vi "tree.vi"(8 "错误输入（无错误）":errorcluster, 11 "search":refnum<vi>) -> (0 "error out":errorcluster, 3 "引用输出":refnum<vi>)   [LabVIEW 2018]
uses:
  Global.vi
  <vilib>/Instr/_visa.llb/VISA Find Search Mode.ctl
panel:
  out "路径":path
  in  "Comunication ports":string(tree)="APMDAQ::0x06"
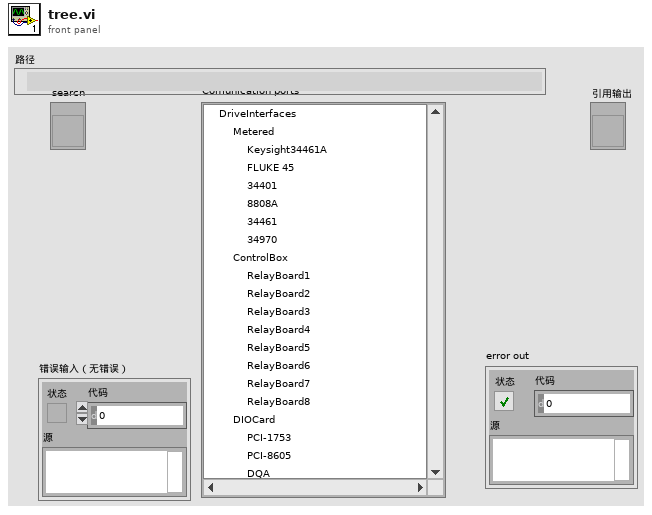
[diagram p1: front panel]
types:
  T1 = enum32{"invalid app kind", "Development System", "Run Time System", "Student Edition", "Embedded LabVIEW", "Evaluation", "Custom"}
  T2 = typedef "imagedata.ctl" = cluster{"image type":i32, "image depth":i32, "image":u8[], "mask":u8[], "colors":u32[], "Rectangle":cluster{"left":i16, "top":i16, "right":i16, "bottom":i16}}
  T3 = typedef "VISA Find Search Mode.ctl" = u32
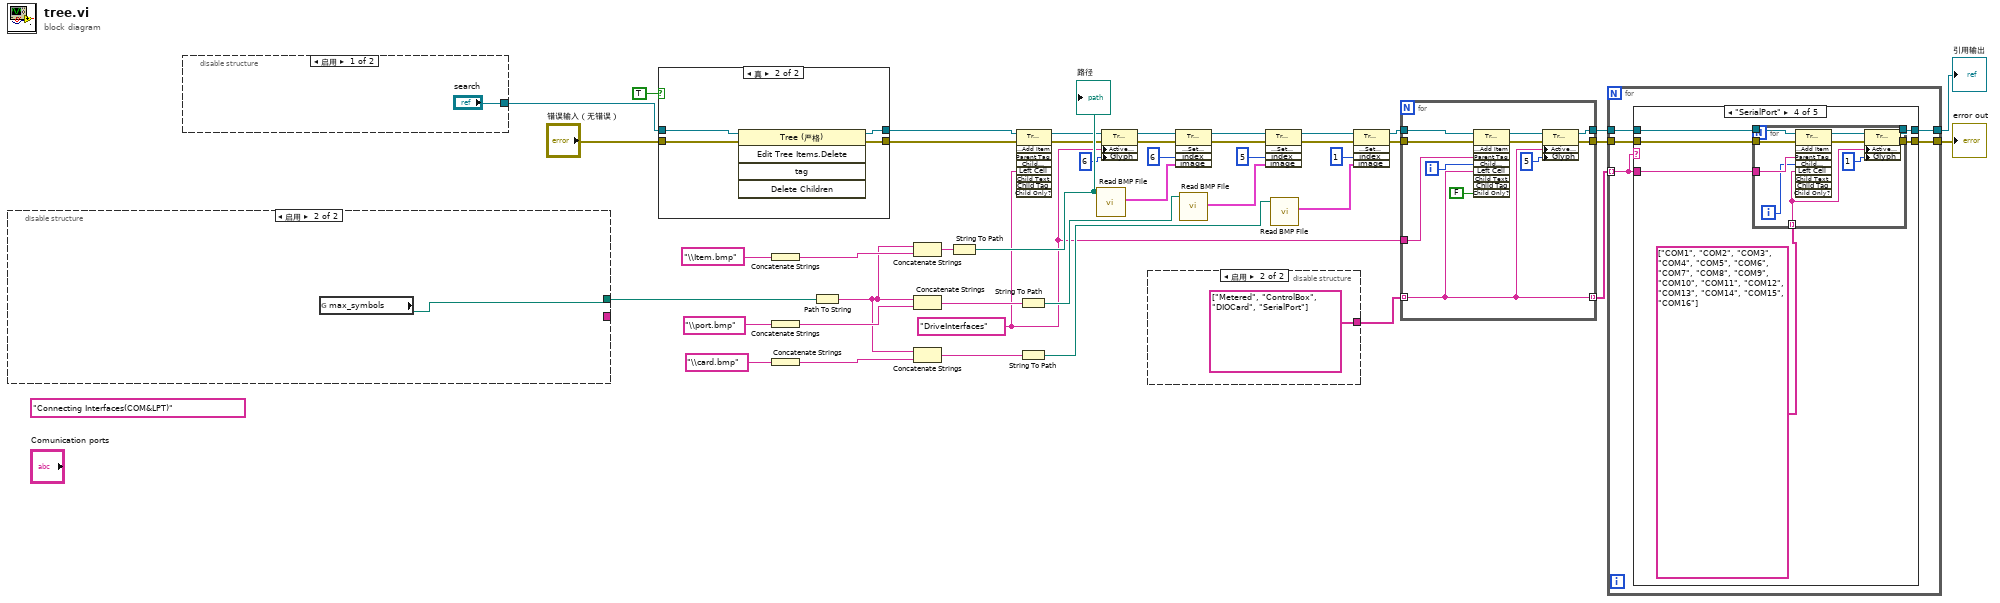
[diagram p0: block diagram]
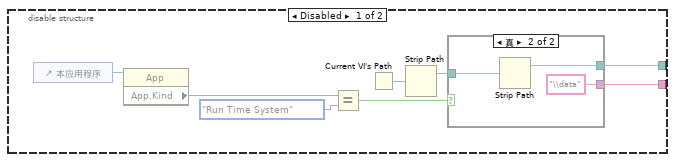
[diagram p2: hidden frame]
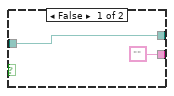
[diagram p3: hidden frame]
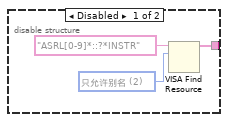
[diagram p4: hidden frame]
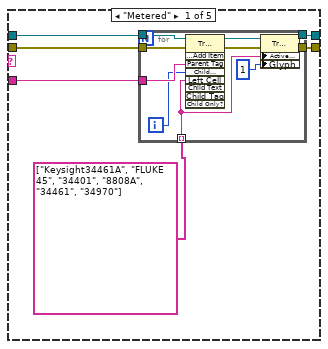
[diagram p5: hidden frame]
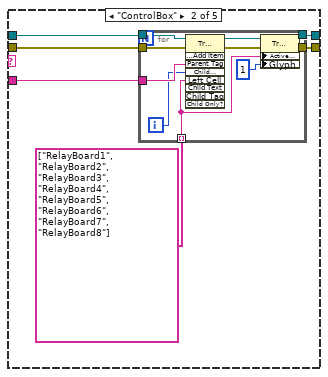
[diagram p6: hidden frame]
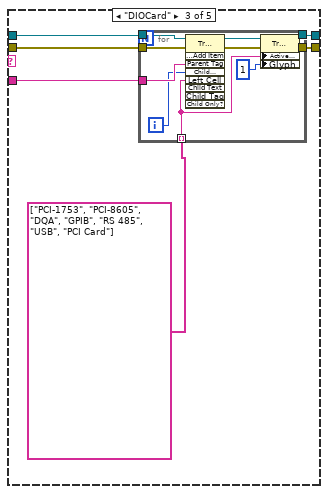
[diagram p7: hidden frame]
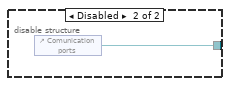
[diagram p10: hidden frame]
diagram:
  w3 = "DriveInterfaces" ("父项标识符")
  (unwired) "Connecting Interfaces(COM&LPT)" ("父项标识符")
  n1 = disable-structure shown="启用" {
    disable-tunnel: [w51 w57] -> w41
    disable-tunnel: [w44 _] -> _
    frame Disabled {
      n2 = control-ref of="本应用程序"() -> (w45:refnum<vi>)
      n3 = property class="App"(reference=w45) -> ("App.Kind"=w46:T1)  [unwired: 1 in, 2 out]
      n4 = Equal?(x=w46, y=T1."Run Time System" ("应用程序:类别")) -> (x = y?=w48:bool)
      n5 = Current VI's Path() -> (path=w49:path)
      n6 = Strip Path(path=w49) -> (stripped path=w50:path)  [unwired: 1 out]
      n7 = case shown="真" w48 {
        tunnel: w50 -> [w53 w56]
        tunnel: [w53 w55] -> w51
        tunnel: ["" "\\data"] -> w44
        frame False {
        }
        frame True {
          n8 = Strip Path(path=w56) -> (stripped path=w55:path)  [unwired: 1 out]
        }
      }
    }
    frame Enabled {
      n9 = global read "Global.vi" "max_symbols"() -> (w57:path)
    }
  }
  n10 = disable-structure shown="启用" {
    disable-tunnel: ["search" w59] -> w35
    frame Enabled {
    }
    frame Disabled {
      n11 = control-ref of="Comunication ports"() -> (w59:refnum<vi>)
    }
  }
  n12 = case shown="真" TRUE {
    tunnel: "错误输入（无错误）" -> [w60 w65]
    tunnel: [w60 w64] -> w37
    tunnel: [w61 w63] -> w22
    tunnel: w35 -> [w61 w62]
    frame False {
    }
    frame True {
      n13 = invoke class="Tree (严格)" method="Edit Tree Items.Delete"(reference=w62, error in=w65) -> (reference out=w63:refnum<vi>, error out=w64:errorcluster)  [unwired: 3 in, 3 out]
    }
  }
  n14 = Concatenate Strings("\\Item.bmp") -> (w33:string)
  n15 = Concatenate Strings("\\port.bmp") -> (w42:string)
  n16 = Concatenate Strings("\\card.bmp") -> (w43:string)
  n17 = Path To String(path=w41) -> (string=w32:string)
  n18 = Concatenate Strings(w32, w33) -> (w31:string)
  n19 = Concatenate Strings(w32, w42) -> (w39:string)
  n20 = Concatenate Strings(w32, w43) -> (w40:string)
  n21 = String To Path(string=w31) -> (path=w23:path)
  "路径" <- w23
  n22 = invoke class="Tree (严格)" method="Edit Tree Items.Add Item"(reference=w22, error in=w37, "Left Cell"=w3) -> (reference out=w18:refnum<vi>, error out=w19:errorcluster)  [unwired: 6 in, 7 out]
  n23 = String To Path(string=w39) -> (path=w27:path)
  n24 = String To Path(string=w40) -> (path=w28:path)
  n25 = call <vilib>:"Read BMP File.vi"("path to BMP file"=w23) -> ("image data"=w24:T2)  [unwired: 1 in, 9 out]
  n26 = property class="Tree (严格)"(reference=w18, error in=w19, "Active Item Tag"=w3, "Glyph"=6 ("活动项:符号索引")) -> (reference out=w8:refnum<vi>, error out=w7:errorcluster)
  n27 = disable-structure shown="启用" {
    disable-tunnel: [w68 string[] ["Metered", "ControlBox", "DIOCard", "SerialPort"] ("find list")] -> w21
    frame Disabled {
      w67 = T3 2 items=["仅允许规范名称"=0, "只允许别名"=2, "包含匹配别名"=3, "包含所有别名"=4] ("Search Mode")
      n28 = VISA Find Resource(10:w67, 11:"ASRL[0-9]*::?*INSTR" ("表达式(\"?*\")")) -> (3:w68:string[])  [unwired: 1 in, 2 out]
    }
    frame Enabled {
    }
  }
  n29 = invoke class="Tree (严格)" method="Custom Item Symbols.Set Symbol"(reference=w8, error in=w7, "index"=6 ("索引"), "image"=w24) -> (reference out=w6:refnum<vi>, error out=w5:errorcluster)  [unwired: 1 in, 3 out]
  n30 = call <vilib>:"Read BMP File.vi"("path to BMP file"=w27) -> ("image data"=w25:T2)  [unwired: 1 in, 9 out]
  n31 = invoke class="Tree (严格)" method="Custom Item Symbols.Set Symbol"(reference=w6, error in=w5, "index"=5 ("索引"), "image"=w25) -> (reference out=w12:refnum<vi>, error out=w13:errorcluster)  [unwired: 1 in, 3 out]
  n32 = call <vilib>:"Read BMP File.vi"("path to BMP file"=w28) -> ("image data"=w26:T2)  [unwired: 1 in, 9 out]
  n33 = invoke class="Tree (严格)" method="Custom Item Symbols.Set Symbol"(reference=w12, error in=w13, "index"=1 ("索引"), "image"=w26) -> (reference out=w14:refnum<vi>, error out=w15:errorcluster)  [unwired: 1 in, 3 out]
  n34 = for {
    tunnel: [w74] -> w11
    tunnel: w3 -> [w79]
    tunnel: w21 -> [w70] mode=indexing
    tunnel: w14 -> [w77]
    tunnel: w15 -> [w76]
    tunnel: [w71] -> w10
    tunnel: [w70] -> w9 mode=indexing
    i -> [w78]
    n35 = invoke class="Tree (严格)" method="Edit Tree Items.Add Item"(reference=w77, error in=w76, "Parent Tag"=w79, "Child Position"=w78, "Left Cell"=w70, "Child Only?"=FALSE ("仅作为子项？")) -> (reference out=w75:refnum<vi>, error out=w73:errorcluster)  [unwired: 3 in, 7 out]
    n36 = property class="Tree (严格)"(reference=w75, error in=w73, "Active Item Tag"=w70, "Glyph"=5 ("活动项:符号索引")) -> (reference out=w74:refnum<vi>, error out=w71:errorcluster)
  }
  n37 = for {
    tunnel: w11 -> [w85]
    tunnel: w10 -> [w84]
    tunnel: w9 -> [w83] mode=indexing
    tunnel: [w82] -> w2
    tunnel: [w81] -> w1
    n38 = case shown="\"SerialPort\"" w83 {
      tunnel: w85 -> [w91 w107 w123 w139 w151]
      tunnel: w84 -> [w90 w106 w122 w138 w150]
      tunnel: w83 -> [w89 w105 w121 w137 _]
      tunnel: [w88 w104 w120 w136 w151] -> w82
      tunnel: [w87 w103 w119 w135 w150] -> w81
      frame "Metered" {
        n39 = for {
          tunnel: w91 -> [w98]
          tunnel: w90 -> [w97]
          tunnel: w89 -> [w96]
          tunnel: [w95] -> w88
          tunnel: [w94] -> w87
          tunnel: string[] ["Keysight34461A", "FLUKE 45", "34401", "8808A", "34461", "34970"] ("find list") -> [w93] mode=indexing
          i -> [w92]
          n40 = invoke class="Tree (严格)" method="Edit Tree Items.Add Item"(reference=w98, error in=w97, "Parent Tag"=w96, "Child Position"=w92, "Left Cell"=w93) -> (reference out=w100:refnum<vi>, error out=w101:errorcluster)  [unwired: 4 in, 7 out]
          n41 = property class="Tree (严格)"(reference=w100, error in=w101, "Active Item Tag"=w93, "Glyph"=1 ("活动项:符号索引")) -> (reference out=w95:refnum<vi>, error out=w94:errorcluster)
        }
      }
      frame "ControlBox" {
        n42 = for {
          tunnel: w107 -> [w114]
          tunnel: w106 -> [w113]
          tunnel: w105 -> [w112]
          tunnel: [w111] -> w104
          tunnel: [w110] -> w103
          tunnel: string[] ["RelayBoard1", "RelayBoard2", "RelayBoard3", "RelayBoard4", "RelayBoard5", "RelayBoard6", "RelayBoard7", "RelayBoard8"] ("find list") -> [w109] mode=indexing
          i -> [w108]
          n43 = invoke class="Tree (严格)" method="Edit Tree Items.Add Item"(reference=w114, error in=w113, "Parent Tag"=w112, "Child Position"=w108, "Left Cell"=w109) -> (reference out=w116:refnum<vi>, error out=w117:errorcluster)  [unwired: 4 in, 7 out]
          n44 = property class="Tree (严格)"(reference=w116, error in=w117, "Active Item Tag"=w109, "Glyph"=1 ("活动项:符号索引")) -> (reference out=w111:refnum<vi>, error out=w110:errorcluster)
        }
      }
      frame "DIOCard" {
        n45 = for {
          tunnel: w123 -> [w130]
          tunnel: w122 -> [w129]
          tunnel: w121 -> [w128]
          tunnel: [w127] -> w120
          tunnel: [w126] -> w119
          tunnel: string[] ["PCI-1753", "PCI-8605", "DQA", "GPIB", "RS 485", "USB", "PCI Card"] ("find list") -> [w125] mode=indexing
          i -> [w124]
          n46 = invoke class="Tree (严格)" method="Edit Tree Items.Add Item"(reference=w130, error in=w129, "Parent Tag"=w128, "Child Position"=w124, "Left Cell"=w125) -> (reference out=w132:refnum<vi>, error out=w133:errorcluster)  [unwired: 4 in, 7 out]
          n47 = property class="Tree (严格)"(reference=w132, error in=w133, "Active Item Tag"=w125, "Glyph"=1 ("活动项:符号索引")) -> (reference out=w127:refnum<vi>, error out=w126:errorcluster)
        }
      }
      frame "SerialPort" {
        n48 = for {
          tunnel: w139 -> [w146]
          tunnel: w138 -> [w145]
          tunnel: w137 -> [w144]
          tunnel: [w143] -> w136
          tunnel: [w142] -> w135
          tunnel: string[] ["COM1", "COM2", "COM3", "COM4", "COM5", "COM6", "COM7", "COM8", "COM9", "COM10", "COM11", "COM12", "COM13", "COM14", "COM15", "COM16"] ("find list") -> [w141] mode=indexing
          i -> [w140]
          n49 = invoke class="Tree (严格)" method="Edit Tree Items.Add Item"(reference=w146, error in=w145, "Parent Tag"=w144, "Child Position"=w140, "Left Cell"=w141) -> (reference out=w148:refnum<vi>, error out=w149:errorcluster)  [unwired: 4 in, 7 out]
          n50 = property class="Tree (严格)"(reference=w148, error in=w149, "Active Item Tag"=w141, "Glyph"=1 ("活动项:符号索引")) -> (reference out=w143:refnum<vi>, error out=w142:errorcluster)
        }
      }
      frame Default {
      }
    }
  }
  "引用输出" <- w2
  "error out" <- w1
